vi "test_read-nmea-data2.vi"() -> ()   [LabVIEW 2019] (continued)
\n15:13:06.78\tF9P\t\t\n15:13:06.80\tF9P\t\t\n15:13:06.82\tF9P\t\t\n15:13:06.84\tF9P\t\t\n15:13:06.86\tF9P\t\t\n15:13:06.88\tF9P\t\t\n15:13:06.90\tF9P\t\t\n15:13:06.92\tF9P\t\t\n15:13:06.94\tF9P\t\t\n15:13:06.96\tF9P\t\t\n15:13:06.98\tF9P\t\t\n15:13:07.00\tF9P\t\t\n15:13:07.02\tF9P\t\t\n15:13:07.04\tF9P\t\t\n15:13:07.06\tF9P\t\t\n15:13:07.08\tF9P\t\t\n15:13:07.10\tF9P\t\t\n15:13:07.12\tF9P\t\t\n15:13:07.14\tF9P\t\t\n15:13:07.16\tF9P\t\t\n15:13:07.18\tF9P\t\t\n15:13:07.20\tF9P\t\t\n15:13:07.22\tF9P\t\t\n15:13:07.24\tF9P\t$GNRMC,061309.00,A,3723.55415,N,12656.97236,E,4.412,80.11,250720,,,A,V*34\n\t\n15:13:07.26\tF9P\t$GNVTG,80.11,T,,M,4.412,N,8.172,K,A*14\n\t\n15:13:07.28\tF9P\t$GNGGA,061309.00,3723.55415,N,12656.97236,E,1,12,0.93,45.1,M,18.5,M,,*70\n\t\n15:13:07.30\tF9P\t$GNGSA,A,3,12,06,19,05,17,09,04,02,,,,,1.63,0.93,1.34,1*08\n\t\n15:13:07.32\tF9P\t$GNGSA,A,3,85,70,71,84,,,,,,,,,1.63,0.93,1.34,2*0A\n\t\n15:13:07.34\tF9P\t$GNGSA,A,3,36,19,11,04,09,12,,,,,,,1.63,0.93,1.34,3*08\n\t\n15:13:07.36\tF9P\t$GNGSA,A,3,14,11,33,,,,,,,,,,1.63,0.93,1.34,4*09\n\t\n15:13:07.38\tF9P\t$GPGSV,3,1,09,02,55,319,22,04,18,043,24,05,37,247,38,06,64,049,35,1*6E\n\t\n15:13:07.40\tF9P\t$GPGSV,3,2,09,09,45,074,33,12,23,276,22,17,33,154,38,19,52,157,32,1*66\n\t\n15:13:07.42\tF9P\t$GPGSV,3,3,09,25,12,306,19,1*54\n\t\n15:13:07.44\tF9P\t$GPGSV,3,1,09,02,55,319,,04,18,043,16,05,37,247,21,06,64,049,30,6*65\n\t\n15:13:07.46\tF9P\t$GPGSV,3,2,09,09,45,074,28,12,23,276,,17,33,154,20,19,52,157,,6*63\n\t\n15:13:07.48\tF9P\t$GPGSV,3,3,09,25,12,306,,6*5B\n\t\n15:13:07.50\tF9P\t$GLGSV,2,1,08,69,11,031,25,70,70,038,20,71,53,206,30,72,05,210,18,1*7D\n\t\n15:13:07.52\tF9P\t$GLGSV,2,2,08,77,01,325,,84,20,122,13,85,70,067,28,86,37,330,,1*73\n\t\n15:13:07.54\tF9P\t$GLGSV,2,1,08,69,11,031,21,70,70,038,,71,53,206,25,72,05,210,,3*74\n\t\n15:13:07.56\tF9P\t$GLGSV,2,2,08,77,01,325,,84,20,122,19,85,70,067,23,86,37,330,,3*70\n\t\n15:13:07.58\tF9P\t$GAGSV,2,1,08,02,08,297,08,04,66,116,29,09,32,193,27,11,72,359,27,7*76\n\t\n15:13:07.60\tF9P\t$GAGSV,2,2,08,12,40,103,28,19,26,045,21,25,09,249,,36,26,308,12,7*72\n\t\n15:13:07.62\tF9P\t$GAGSV,2,1,08,02,08,297,,04,66,116,,09,32,193,,11,72,359,,2*70\n\t\n15:13:07.64\tF9P\t$GAGSV,2,2,08,12,40,103,,19,26,045,,25,09,249,,36,26,308,,2*7D\n\t\n15:13:07.66\tF9P\t$GBGSV,1,1,04,11,49,132,27,14,87,114,23,28,,,21,33,61,220,35,1*4D\n\t\n15:13:07.68\tF9P\t$GBGSV,1,1,03,11,49,132,29,14,87,114,,33,61,220,,3*48\n\t\n15:13:07.70\tF9P\t$GNGLL,3723.55415,N,12656.97236,E,061309.00,A,A*70\n\t\n15:13:07.72\tF9P\t\t\n15:13:07.74\tF9P\t\t\n15:13:07.76\tF9P\t\t\n15:13:07.78\tF9P\t\t\n15:13:07.80\tF9P\t\t\n15:13:07.82\tF9P\t\t\n15:13:07.84\tF9P\t\t\n15:13:07.86\tF9P\t\t\n15:13:07.88\tF9P\t\t\n15:13:07.90\tF9P\t\t\n15:13:07.92\tF9P\t\t\n15:13:07.94\tF9P\t\t\n15:13:07.96\tF9P\t\t\n15:13:07.98\tF9P\t\t\n15:13:08.00\tF9P\t\t\n15:13:08.02\tF9P\t\t\n15:13:08.04\tF9P\t\t\n15:13:08.06\tF9P\t\t\n15:13:08.08\tF9P\t\t\n15:13:08.10\tF9P\t\t\n15:13:08.12\tF9P\t\t\n15:13:08.14\tF9P\t\t\n15:13:08.16\tF9P\t\t\n15:13:08.18\tF9P\t\t\n15:13:08.20\tF9P\t\t\n15:13:08.22\tF9P\t\t\n15:13:08.24\tF9P\t$GNRMC,061310.00,A,3723.55430,N,12656.97323,E,2.033,80.21,250720,,,A,V*3C\n\t\n15:13:08.26\tF9P\t$GNVTG,80.21,T,,M,2.033,N,3.766,K,A*1E\n\t\n15:13:08.28\tF9P\t$GNGGA,061310.00,3723.55430,N,12656.97323,E,1,12,0.86,46.0,M,18.5,M,,*7C\n\t\n15:13:08.30\tF9P\t$GNGSA,A,3,12,06,19,05,17,09,04,02,,,,,1.43,0.86,1.13,1*0B\n\t\n15:13:08.32\tF9P\t$GNGSA,A,3,85,70,71,84,,,,,,,,,1.43,0.86,1.13,2*09\n\t\n15:13:08.34\tF9P\t$GNGSA,A,3,36,19,11,04,09,12,,,,,,,1.43,0.86,1.13,3*0B\n\t\n15:13:08.36\tF9P\t$GNGSA,A,3,14,11,33,,,,,,,,,,1.43,0.86,1.13,4*0A\n\t\n15:13:08.38\tF9P\t$GPGSV,3,1,09,02,55,319,22,04,18,043,23,05,37,247,32,06,64,049,34,1*62\n\t\n15:13:08.40\tF9P\t$GPGSV,3,2,09,09,45,074,34,12,23,276,20,17,33,154,32,19,52,157,34,1*6F\n\t\n15:13:08.42\tF9P\t$GPGSV,3,3,09,25,12,306,18,1*55\n\t\n15:13:08.44\tF9P\t$GPGSV,3,1,09,02,55,319,,04,18,043,14,05,37,247,22,06,64,049,23,6*66\n\t\n15:13:08.46\tF9P\t$GPGSV,3,2,09,09,45,074,28,12,23,276,,17,33,154,22,19,52,157,,6*61\n\t\n15:13:08.48\tF9P\t$GPGSV,3,3,09,25,12,306,,6*5B\n\t\n15:13:08.50\tF9P\t$GLGSV,2,1,08,69,11,031,24,70,70,038,24,71,53,206,29,72,05,210,19,1*71\n\t\n15:13:08.52\tF9P\t$GLGSV,2,2,08,77,01,325,,84,20,122,09,85,70,067,28,86,37,330,,1*78\n\t\n15:13:08.54\tF9P\t$GLGSV,2,1,08,69,11,031,19,70,70,038,,71,53,206,25,72,05,210,,3*7F\n\t\n15:13:08.56\tF9P\t$GLGSV,2,2,08,77,01,325,,84,20,122,19,85,70,067,22,86,37,330,,3*71\n\t\n15:13:08.58\tF9P\t$GAGSV,2,1,08,02,08,297,09,04,66,116,30,09,32,193,26,11,72,359,32,7*7A\n\t\n15:13:08.60\tF9P\t$GAGSV,2,2,08,12,40,103,29,19,26,045,21,25,09,249,,36,26,308,12,7*73\n\t\n15:13:08.62\tF9P\t$GAGSV,2,1,08,02,08,297,,04,66,116,29,09,32,193,,11,72,359,,2*7B\n\t\n15:13:08.64\tF9P\t$GAGSV,2,2,08,12,40,103,,19,26,045,,25,09,249,,36,26,308,,2*7D\n\t\n15:13:08.66\tF9P\t$GBGSV,1,1,04,11,49,132,31,14,87,114,26,28,,,21,33,61,220,31,1*4B\n\t\n15:13:08.68\tF9P\t$GBGSV,1,1,03,11,49,132,32,14,87,114,,33,61,220,,3*42\n\t\n15:13:08.70\tF9P\t$GNGLL,3723.55430,N,12656.97323,E,061310.00,A,A*7A\n\t\n15:13:08.72\tF9P\t\t\n15:13:08.74\tF9P\t\t\n15:13:08.76\tF9P\t\t\n15:13:08.78\tF9P\t\t\n15:13:08.80\tF9P\t\t\n15:13:08.82\tF9P\t\t\n15:13:08.84\tF9P\t\t\n15:13:08.86\tF9P\t\t\n15:13:08.88\tF9P\t\t\n15:13:08.90\tF9P\t\t\n15:13:08.92\tF9P\t\t\n15:13:08.94\tF9P\t\t\n15:13:08.96\tF9P\t\t\n15:13:08.98\tF9P\t\t\n15:13:09.00\tF9P\t\t\n15:13:09.02\tF9P\t\t\n15:13:09.04\tF9P\t\t\n15:13:09.06\tF9P\t\t\n15:13:09.08\tF9P\t\t\n15:13:09.10\tF9P\t\t\n15:13:09.12\tF9P\t\t\n15:13:09.14\tF9P\t\t\n15:13:09.16\tF9P\t\t\n15:13:09.18\tF9P\t\t\n15:13:09.20\tF9P\t\t\n15:13:09.22\tF9P\t\t\n15:13:09.24\tF9P\t$GNRMC,061311.00,A,3723.55466,N,12656.97390,E,2.064,69.29,250720,,,A,V*3B\n\t\n15:13:09.26\tF9P\t$GNVTG,69.29,T,,M,2.064,N,3.823,K,A*1D\n\t\n15:13:09.28\tF9P\t$GNGGA,061311.00,3723.55466,N,12656.97390,E,1,12,0.86,46.4,M,18.5,M,,*72\n\t\n15:13:09.30\tF9P\t$GNGSA,A,3,12,06,19,05,17,09,04,02,,,,,1.43,0.86,1.13,1*0B\n\t\n15:13:09.32\tF9P\t$GNGSA,A,3,85,70,71,84,,,,,,,,,1.43,0.86,1.13,2*09\n\t\n15:13:09.34\tF9P\t$GNGSA,A,3,19,11,04,09,12,,,,,,,,1.43,0.86,1.13,3*0E\n\t\n15:13:09.36\tF9P\t$GNGSA,A,3,14,11,33,,,,,,,,,,1.43,0.86,1.13,4*0A\n\t\n15:13:09.38\tF9P\t$GPGSV,3,1,09,02,55,319,21,04,18,043,22,05,37,247,30,06,64,049,30,1*66\n\t\n15:13:09.40\tF9P\t$GPGSV,3,2,09,09,45,074,30,12,23,276,20,17,33,154,35,19,52,157,30,1*68\n\t\n15:13:09.42\tF9P\t$GPGSV,3,3,09,25,12,306,19,1*54\n\t\n15:13:09.44\tF9P\t$GPGSV,3,1,09,02,55,319,,04,18,043,14,05,37,247,21,06,64,049,22,6*64\n\t\n15:13:09.46\tF9P\t$GPGSV,3,2,09,09,45,074,19,12,23,276,,17,33,154,25,19,52,157,,6*64\n\t\n15:13:09.48\tF9P\t$GPGSV,3,3,09,25,12,306,,6*5B\n\t\n15:13:09.50\tF9P\t$GLGSV,2,1,08,69,11,031,24,70,70,038,24,71,53,206,34,72,05,210,22,1*75\n\t\n15:13:09.52\tF9P\t$GLGSV,2,2,08,77,01,325,,84,20,122,15,85,70,067,28,86,37,330,,1*75\n\t\n15:13:09.54\tF9P\t$GLGSV,2,1,08,69,11,031,18,70,70,038,,71,53,206,27,72,05,210,,3*7C\n\t\n15:13:09.56\tF9P\t$GLGSV,2,2,08,77,01,325,,84,20,122,18,85,70,067,21,86,37,330,,3*73\n\t\n15:13:09.58\tF9P\t$GAGSV,2,1,08,02,08,297,10,04,66,116,29,09,32,193,32,11,72,359,35,7*78\n\t\n15:13:09.60\tF9P\t$GAGSV,2,2,08,12,40,103,27,19,26,045,19,25,09,249,,36,26,308,10,7*74\n\t\n15:13:09.62\tF9P\t$GAGSV,2,1,08,02,08,297,,04,66,116,,09,32,193,,11,72,359,,2*70\n\t\n15:13:09.64\tF9P\t$GAGSV,2,2,08,12,40,103,,19,26,045,,25,09,249,,36,26,308,,2*7D\n\t\n15:13:09.66\tF9P\t$GBGSV,1,1,04,11,49,132,30,14,87,114,30,28,,,21,33,61,220,35,1*49\n\t\n15:13:09.68\tF9P\t$GBGSV,1,1,03,11,49,132,28,14,87,114,,33,61,220,,3*49\n\t\n15:13:09.70\tF9P\t$GNGLL,3723.55466,N,12656.97390,E,061311.00,A,A*70\n\t\n15:13:09.72\tF9P\t\t\n15:13:09.74\tF9P\t\t\n15:13:09.76\tF9P\t\t\n15:13:09.78\tF9P\t\t\n15:13:09.80\tF9P\t\t\n15:13:09.82\tF9P\t\t\n15:13:09.84\tF9P\t\t\n15:13:09.86\tF9P\t\t\n15:13:09.88\tF9P\t\t\n15:13:09.90\tF9P\t\t\n15:13:09.92\tF9P\t\t\n15:13:09.94\tF9P\t\t\n15:13:09.96\tF9P\t\t\n15:13:09.98\tF9P\t\t\n15:13:10.00\tF9P\t\t\n15:13:10.02\tF9P\t\t\n15:13:10.04\tF9P\t\t\n15:13:10.06\tF9P\t\t\n15:13:10.08\tF9P\t\t\n15:13:10.10\tF9P\t\t\n15:13:10.12\tF9P\t\t\n15:13:10.14\tF9P\t\t\n15:13:10.16\tF9P\t\t\n15:13:10.18\tF9P\t\t\n15:13:10.20\tF9P\t\t\n15:13:10.22\tF9P\t\t\n15:13:10.24\tF9P\t$GNRMC,061312.00,A,3723.55500,N,12656.97464,E,2.191,68.08,250720,,,A,V*3C\n\t\n15:13:10.26\tF9P\t$GNVTG,68.08,T,,M,2.191,N,4.057,K,A*18\n\t\n15:13:10.28\tF9P\t$GNGGA,061312.00,3723.55500,N,12656.97464,E,1,12,0.86,46.1,M,18.5,M,,*79\n\t\n15:13:10.30\tF9P\t$GNGSA,A,3,12,06,19,05,17,09,04,02,,,,,1.43,0.86,1.13,1*0B\n\t\n15:13:10.32\tF9P\t$GNGSA,A,3,85,70,71,84,,,,,,,,,1.43,0.86,1.13,2*09\n\t\n15:13:10.34\tF9P\t$GNGSA,A,3,36,19,11,04,09,12,,,,,,,1.43,0.86,1.13,3*0B\n\t\n15:13:10.36\tF9P\t$GNGSA,A,3,14,11,33,,,,,,,,,,1.43,0.86,1.13,4*0A\n\t\n15:13:10.38\tF9P\t$GPGSV,3,1,09,02,55,319,22,04,18,043,25,05,37,247,31,06,64,049,33,1*60\n\t\n15:13:10.40\tF9P\t$GPGSV,3,2,09,09,45,074,30,12,23,276,21,17,33,154,30,19,52,157,30,1*6C\n\t\n15:13:10.42\tF9P\t$GPGSV,3,3,09,25,12,306,18,1*55\n\t\n15:13:10.44\tF9P\t$GPGSV,3,1,09,02,55,319,,04,18,043,14,05,37,247,21,06,64,049,21,6*67\n\t\n15:13:10.46\tF9P\t$GPGSV,3,2,09,09,45,074,24,12,23,276,,17,33,154,24,19,52,157,,6*6B\n\t\n15:13:10.48\tF9P\t$GPGSV,3,3,09,25,12,306,,6*5B\n\t\n15:13:10.50\tF9P\t$GLGSV,2,1,08,69,11,031,22,70,70,038,22,71,53,206,44,72,05,210,22,1*72\n\t\n15:13:10.52\tF9P\t$GLGSV,2,2,08,77,01,325,,84,20,122,14,85,70,067,28,86,37,330,,1*74\n\t\n15:13:10.54\tF9P\t$GLGSV,2,1,08,69,11,031,15,70,70,038,,71,53,206,27,72,05,210,,3*71\n\t\n15:13:10.56\tF9P\t$GLGSV,2,2,08,77,01,325,,84,20,122,18,85,70,067,21,86,37,330,,3*73\n\t\n15:13:10.58\tF9P\t$GAGSV,2,1,08,02,08,297,07,04,66,116,28,09,32,193,28,11,72,359,28,7*78\n\t\n15:13:10.60\tF9P\t$GAGSV,2,2,08,12,40,103,31,19,26,045,18,25,09,249,,36,26,308,14,7*76\n\t\n15:13:10.62\tF9P\t$GAGSV,2,1,08,02,08,297,,04,66,116,27,09,32,193,,11,72,359,,2*75\n\t\n15:13:10.64\tF9P\t$GAGSV,2,2,08,12,40,103,,19,26,045,,25,09,249,,36,26,308,,2*7D\n\t\n15:13:10.66\tF9P\t$GBGSV,1,1,04,11,49,132,29,14,87,114,29,28,,,22,33,61,220,38,1*47\n\t\n15:13:10.68\tF9P\t$GBGSV,1,1,03,11,49,132,27,14,87,114,,33,61,220,,3*46\n\t\n15:13:10.70\tF9P\t$GNGLL,3723.55500,N,12656.97464,E,061312.00,A,A*7E\n\t\n15:13:10.72\tF9P\t\t\n15:13:10.74\tF9P\t\t\n15:13:10.76\tF9P\t\t\n15:13:10.78\tF9P\t\t\n15:13:10.80\tF9P\t\t\n15:13:10.82\tF9P\t\t\n15:13:10.84\tF9P\t\t\n15:13:10.86\tF9P\t\t\n15:13:10.88\tF9P\t\t\n15:13:10.90\tF9P\t\t\n15:13:10.92\tF9P\t\t\n15:13:10.94\tF9P\t\t\n15:13:10.96\tF9P\t\t\n15:13:10.98\tF9P\t\t\n15:13:11.00\tF9P\t\t\n15:13:11.02\tF9P\t\t\n15:13:11.04\tF9P\t\t\n15:13:11.06\tF9P\t\t\n15:13:11.08\tF9P\t\t\n15:13:11.10\tF9P\t\t\n15:13:11.12\tF9P\t\t\n15:13:11.14\tF9P\t\t\n15:13:11.16\tF9P\t\t\n15:13:11.18\tF9P\t\t\n15:13:11.20\tF9P\t\t\n15:13:11.22\tF9P\t\t\n15:13:11.24\tF9P\t$GNRMC,061313.00,A,3723.55544,N,12656.97538,E,2.422,61.28,250720,,,A,V*33\n\t\n15:13:11.26\tF9P\t$GNVTG,61.28,T,,M,2.422,N,4.486,K,A*16\n\t\n15:13:11.28\tF9P\t$GNGGA,061313.00,3723.55544,N,12656.97538,E,1,12,0.91,46.4,M,18.5,M,,*73\n\t\n15:13:11.30\tF9P\t$GNGSA,A,3,12,06,19,05,17,09,04,02,,,,,1.51,0.91,1.20,1*0E\n\t\n15:13:11.32\tF9P\t$GNGSA,A,3,85,70,71,84,,,,,,,,,1.51,0.91,1.20,2*0C\n\t\n15:13:11.34\tF9P\t$GNGSA,A,3,36,19,11,04,09,12,,,,,,,1.51,0.91,1.20,3*0E\n\t\n15:13:11.36\tF9P\t$GNGSA,A,3,14,11,33,,,,,,,,,,1.51,0.91,1.20,4*0F\n\t\n15:13:11.38\tF9P\t$GPGSV,3,1,09,02,55,319,22,04,18,043,25,05,37,247,32,06,64,049,34,1*64\n\t\n15:13:11.40\tF9P\t$GPGSV,3,2,09,09,45,074,24,12,23,276,21,17,33,154,34,19,52,157,35,1*68\n\t\n15:13:11.42\tF9P\t$GPGSV,3,3,09,25,12,306,17,1*5A\n\t\n15:13:11.44\tF9P\t$GPGSV,3,1,09,02,55,319,,04,18,043,15,05,37,247,20,06,64,049,21,6*67\n\t\n15:13:11.46\tF9P\t$GPGSV,3,2,09,09,45,074,27,12,23,276,,17,33,154,22,19,52,157,,6*6E\n\t\n15:13:11.48\tF9P\t$GPGSV,3,3,09,25,12,306,,6*5B\n\t\n15:13:11.50\tF9P\t$GLGSV,2,1,08,69,11,031,23,70,70,038,23,71,53,206,36,72,05,210,20,1*75\n\t\n15:13:11.52\tF9P\t$GLGSV,2,2,08,77,01,325,,84,19,123,11,85,70,067,28,86,37,330,,1*7A\n\t\n15:13:11.54\tF9P\t$GLGSV,2,1,08,69,11,031,17,70,70,038,,71,53,206,27,72,05,210,,3*73\n\t\n15:13:11.56\tF9P\t$GLGSV,2,2,08,77,01,325,,84,19,123,19,85,70,067,22,86,37,330,,3*7A\n\t\n15:13:11.58\tF9P\t$GAGSV,2,1,08,02,08,297,10,04,66,116,33,09,32,193,26,11,72,359,32,7*71\n\t\n15:13:11.60\tF9P\t$GAGSV,2,2,08,12,40,103,30,19,26,045,17,25,09,249,,36,26,308,16,7*7A\n\t\n15:13:11.62\tF9P\t$GAGSV,2,1,08,02,08,297,,04,66,116,35,09,32,193,,11,72,359,,2*76\n\t\n15:13:11.64\tF9P\t$GAGSV,2,2,08,12,40,103,,19,26,045,,25,09,249,,36,26,308,,2*7D\n\t\n15:13:11.66\tF9P\t$GBGSV,1,1,04,11,49,132,30,14,87,114,23,28,,,23,33,61,220,33,1*4F\n\t\n15:13:11.68\tF9P\t$GBGSV,1,1,03,11,49,132,28,14,87,114,,33,61,220,,3*49\n\t\n15:13:11.70\tF9P\t$GNGLL,3723.55544,N,12656.97538,E,061313.00,A,A*77\n\t\n15:13:11.72\tF9P\t\t\n15:13:11.74\tF9P\t\t\n15:13:11.76\tF9P\t\t\n15:13:11.78\tF9P\t\t\n15:13:11.80\tF9P\t\t\n15:13:11.82\tF9P\t\t\n15:13:11.84\tF9P\t\t\n15:13:11.86\tF9P\t\t\n15:13:11.88\tF9P\t\t\n15:13:11.90\tF9P\t\t\n15:13:11.92\tF9P\t\t\n15:13:11.94\tF9P\t\t\n15:13:11.96\tF9P\t\t\n15:13:11.98\tF9P\t\t\n15:13:12.00\tF9P\t\t\n15:13:12.02\tF9P\t\t\n15:13:12.04\tF9P\t\t\n15:13:12.06\tF9P\t\t\n15:13:12.08\tF9P\t\t\n15:13:12.10\tF9P\t\t\n15:13:12.12\tF9P\t\t\n15:13:12.14\tF9P\t\t\n15:13:12.16\tF9P\t\t\n15:13:12.18\tF9P\t\t\n15:13:12.20\tF9P\t\t\n15:13:12.22\tF9P\t\t\n15:13:12.24\tF9P\t$GNRMC,061314.00,A,3723.55582,N,12656.97605,E,1.937,55.76,250720,,,A,V*35\n\t\n15:13:12.26\tF9P\t$GNVTG,55.76,T,,M,1.937,N,3.588,K,A*18\n\t\n15:13:12.28\tF9P\t$GNGGA,061314.00,3723.55582,N,12656.97605,E,1,12,0.86,47.2,M,18.5,M,,*72\n\t\n15:13:12.30\tF9P\t$GNGSA,A,3,12,06,19,05,17,09,04,02,,,,,1.43,0.86,1.13,1*0B\n\t\n15:13:12.32\tF9P\t$GNGSA,A,3,85,70,71,84,,,,,,,,,1.43,0.86,1.13,2*09\n\t\n15:13:12.34\tF9P\t$GNGSA,A,3,36,19,11,04,09,12,,,,,,,1.43,0.86,1.13,3*0B\n\t\n15:13:12.36\tF9P\t$GNGSA,A,3,14,11,33,,,,,,,,,,1.43,0.86,1.13,4*0A\n\t\n15:13:12.38\tF9P\t$GPGSV,3,1,09,02,55,319,23,04,18,043,24,05,37,247,33,06,64,049,30,1*61\n\t\n15:13:12.40\tF9P\t$GPGSV,3,2,09,09,45,074,30,12,23,276,21,17,33,154,36,19,52,157,29,1*62\n\t\n15:13:12.42\tF9P\t$GPGSV,3,3,09,25,12,306,17,1*5A\n\t\n15:13:12.44\tF9P\t$GPGSV,3,1,09,02,55,319,,04,18,043,15,05,37,247,21,06,64,049,23,6*64\n\t\n15:13:12.46\tF9P\t$GPGSV,3,2,09,09,45,074,27,12,23,276,,17,33,154,23,19,52,157,,6*6F\n\t\n15:13:12.48\tF9P\t$GPGSV,3,3,09,25,12,306,,6*5B\n\t\n15:13:12.50\tF9P\t$GLGSV,2,1,08,69,11,031,23,70,70,038,25,71,53,206,30,72,05,210,21,1*74\n\t\n15:13:12.52\tF9P\t$GLGSV,2,2,08,77,01,325,,84,19,123,11,85,70,070,28,86,37,330,,1*7C\n\t\n15:13:12.54\tF9P\t$GLGSV,2,1,08,69,11,031,17,70,70,038,,71,53,206,26,72,05,210,,3*72\n\t\n15:13:12.56\tF9P\t$GLGSV,2,2,08,77,01,325,,84,19,123,19,85,70,070,21,86,37,330,,3*7F\n\t\n15:13:12.58\tF9P\t$GAGSV,2,1,08,02,08,297,10,04,66,116,29,09,32,193,33,11,72,359,26,7*7B\n\t\n15:13:12.60\tF9P\t$GAGSV,2,2,08,12,40,103,32,19,26,045,18,25,09,249,,36,26,308,16,7*77\n\t\n15:13:12.62\tF9P\t$GAGSV,2,1,08,02,08,297,,04,66,116,32,09,32,193,,11,72,359,,2*71\n\t\n15:13:12.64\tF9P\t$GAGSV,2,2,08,12,40,103,29,19,26,045,,25,09,249,,36,26,308,,2*76\n\t\n15:13:12.66\tF9P\t$GBGSV,1,1,04,11,49,132,34,14,87,114,23,28,,,22,33,61,220,36,1*4F\n\t\n15:13:12.68\tF9P\t$GBGSV,1,1,03,11,49,132,32,14,87,114,,33,61,220,,3*42\n\t\n15:13:12.70\tF9P\t$GNGLL,3723.55582,N,12656.97605,E,061314.00,A,A*77\n\t\n15:13:12.72\tF9P\t\t\n15:13:12.74\tF9P\t\t\n15:13:12.76\tF9P\t\t\n15:13:12.78\tF9P\t\t\n15:13:12.80\tF9P\t\t\n15:13:12.82\tF9P\t\t\n15:13:12.84\tF9P\t\t\n15:13:12.86\tF9P\t\t\n15:13:12.88\tF9P\t\t\n15:13:12.90\tF9P\t\t\n15:13:12.92\tF9P\t\t\n15:13:12.94\tF9P\t\t\n15:13:12.96\tF9P\t\t\n15:13:12.98\tF9P\t\t\n15:13:13.00\tF9P\t\t\n15:13:13.02\tF9P\t\t\n15:13:13.04\tF9P\t\t\n15:13:13.06\tF9P\t\t\n15:13:13.08\tF9P\t\t\n15:13:13.10\tF9P\t\t\n15:13:13.12\tF9P\t\t\n15:13:13.14\tF9P\t\t\n15:13:13.16\tF9P\t\t\n15:13:13.18\tF9P\t\t\n15:13:13.20\tF9P\t\t\n15:13:13.22\tF9P\t\t\n15:13:13.24\tF9P\t$GNRMC,061315.00,A,3723.55611,N,12656.97670,E,2.039,43.98,250720,,,A,V*3C\n\t\n15:13:13.26\tF9P\t$GNVTG,43.98,T,,M,2.039,N,3.777,K,A*19\n\t\n15:13:13.28\tF9P\t$GNGGA,061315.00,3723.55611,N,12656.97670,E,1,12,0.86,48.9,M,18.5,M,,*7C\n\t\n15:13:13.30\tF9P\t$GNGSA,A,3,12,06,19,05,17,09,04,02,,,,,1.43,0.86,1.13,1*0B\n\t\n15:13:13.32\tF9P\t$GNGSA,A,3,85,70,71,84,,,,,,,,,1.43,0.86,1.13,2*09\n\t\n15:13:13.34\tF9P\t$GNGSA,A,3,36,19,11,04,09,12,,,,,,,1.43,0.86,1.13,3*0B\n\t\n15:13:13.36\tF9P\t$GNGSA,A,3,14,11,33,,,,,,,,,,1.43,0.86,1.13,4*0A\n\t\n15:13:13.38\tF9P\t$GPGSV,3,1,09,02,55,319,23,04,18,043,23,05,37,247,42,06,64,049,26,1*67\n\t\n15:13:13.40\tF9P\t$GPGSV,3,2,09,09,45,074,30,12,23,276,22,17,33,154,40,19,52,157,29,1*60\n\t\n15:13:13.42\tF9P\t$GPGSV,3,3,09,25,12,306,18,1*55\n\t\n15:13:13.44\tF9P\t$GPGSV,3,1,09,02,55,319,,04,18,043,17,05,37,247,22,06,64,049,24,6*62\n\t\n15:13:13.46\tF9P\t$GPGSV,3,2,09,09,45,074,28,12,23,276,,17,33,154,24,19,52,157,,6*67\n\t\n15:13:13.48\tF9P\t$GPGSV,3,3,09,25,12,306,,6*5B\n\t\n15:13:13.50\tF9P\t$GLGSV,2,1,08,69,11,031,25,70,70,038,25,71,53,206,33,72,05,210,21,1*71\n\t\n15:13:13.52\tF9P\t$GLGSV,2,2,08,77,01,325,,84,19,123,10,85,70,070,28,86,37,330,,1*7D\n\t\n15:13:13.54\tF9P\t$GLGSV,2,1,08,69,11,031,15,70,70,038,,71,53,206,26,72,05,210,,3*70\n\t\n15:13:13.56\tF9P\t$GLGSV,2,2,08,77,01,325,,84,19,123,19,85,70,070,20,86,37,330,,3*7E\n\t\n15:13:13.58\tF9P\t$GAGSV,2,1,08,02,08,297,10,04,66,116,30,09,32,193,32,11,72,359,33,7*76\n\t\n15:13:13.60\tF9P\t$GAGSV,2,2,08,12,40,103,30,19,26,045,19,25,09,249,,36,26,308,16,7*74\n\t\n15:13:13.62\tF9P\t$GAGSV,2,1,08,02,08,297,,04,66,116,31,09,32,193,,11,72,359,,2*72\n\t\n15:13:13.64\tF9P\t$GAGSV,2,2,08,12,40,103,,19,26,045,,25,09,249,,36,26,308,,2*7D\n\t\n15:13:13.66\tF9P\t$GBGSV,1,1,04,11,49,132,31,14,87,114,30,28,,,21,33,61,220,31,1*4C\n\t\n15:13:13.68\tF9P\t$GBGSV,1,1,03,11,49,132,,14,87,114,,33,61,220,,3*43\n\t\n15:13:13.70\tF9P\t$GNGLL,3723.55611,N,12656.97670,E,061315.00,A,A*7D\n\t\n15:13:13.72\tF9P\t\t\n15:13:13.74\tF9P\t\t\n15:13:13.76\tF9P\t\t\n15:13:13.78\tF9P\t\t\n15:13:13.80\tF9P\t\t\n15:13:13.82\tF9P\t\t\n15:13:13.84\tF9P\t\t\n15:13:13.86\tF9P\t\t\n15:13:13.88\tF9P\t\t\n15:13:13.90\tF9P\t\t\n15:13:13.92\tF9P\t\t\n15:13:13.94\tF9P\t\t\n15:13:13.96\tF9P\t\t\n15:13:13.98\tF9P\t\t\n15:13:14.00\tF9P\t\t\n15:13:14.02\tF9P\t\t\n15:13:14.04\tF9P\t\t\n15:13:14.06\tF9P\t\t\n15:13:14.08\tF9P\t\t\n15:13:14.10\tF9P\t\t\n15:13:14.12\tF9P\t\t\n15:13:14.14\tF9P\t\t\n15:13:14.16\tF9P\t\t\n15:13:14.18\tF9P\t\t\n15:13:14.20\tF9P\t\t\n15:13:14.22\tF9P\t\t\n15:13:14.24\tF9P\t$GNRMC,061316.00,A,3723.55651,N,12656.97723,E,1.759,42.83,250720,,,A,V*35\n\t\n15:13:14.26\tF9P\t$GNVTG,42.83,T,,M,1.759,N,3.257,K,A*17\n\t\n15:13:14.28\tF9P\t$GNGGA,061316.00,3723.55651,N,12656.97723,E,1,12,0.86,49.8,M,18.5,M,,*7C\n\t\n15:13:14.30\tF9P\t$GNGSA,A,3,12,06,19,05,17,09,04,02,,,,,1.43,0.86,1.13,1*0B\n\t\n15:13:14.32\tF9P\t$GNGSA,A,3,85,70,71,84,,,,,,,,,1.43,0.86,1.13,2*09\n\t\n15:13:14.34\tF9P\t$GNGSA,A,3,36,19,11,04,09,12,,,,,,,1.43,0.86,1.13,3*0B\n\t\n15:13:14.36\tF9P\t$GNGSA,A,3,14,11,33,,,,,,,,,,1.43,0.86,1.13,4*0A\n\t\n15:13:14.38\tF9P\t$GPGSV,3,1,09,02,55,319,22,04,18,043,23,05,37,247,37,06,64,049,31,1*62\n\t\n15:13:14.40\tF9P\t$GPGSV,3,2,09,09,45,074,30,12,23,276,22,17,33,154,30,19,52,157,33,1*6C\n\t\n15:13:14.42\tF9P\t$GPGSV,3,3,09,25,12,306,20,1*5E\n\t\n15:13:14.44\tF9P\t$GPGSV,3,1,09,02,55,319,,04,18,043,17,05,37,247,23,06,64,049,29,6*6E\n\t\n15:13:14.46\tF9P\t$GPGSV,3,2,09,09,45,074,29,12,23,276,,17,33,154,23,19,52,157,,6*61\n\t\n15:13:14.48\tF9P\t$GPGSV,3,3,09,25,12,306,,6*5B\n\t\n15:13:14.50\tF9P\t$GLGSV,2,1,08,69,11,031,26,70,70,038,25,71,53,206,38,72,05,210,23,1*7B\n\t\n15:13:14.52\tF9P\t$GLGSV,2,2,08,77,01,325,,84,19,123,13,85,70,070,28,86,37,330,,1*7E\n\t\n15:13:14.54\tF9P\t$GLGSV,2,1,08,69,11,031,27,70,70,038,,71,53,206,31,72,05,210,,3*77\n\t\n15:13:14.56\tF9P\t$GLGSV,2,2,08,77,01,325,,84,19,123,20,85,70,070,19,86,37,330,,3*7E\n\t\n15:13:14.58\tF9P\t$GAGSV,2,1,08,02,08,297,11,04,66,116,24,09,32,193,32,
